vi "FormatLength.vi"(10 "length":i32) -> (2 "encoded length":string)   [LabVIEW 2014, in "Raspberry Pi Compatible Compiler for LabVIEW.lvlib" / "Websocket.lvlib"]
uses:
  Websocket.lvlib
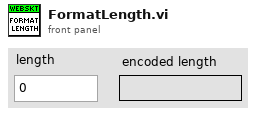
[diagram p1: front panel]
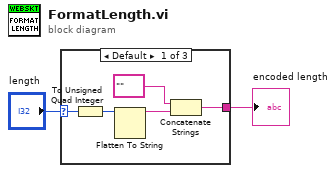
[diagram p0: block diagram]
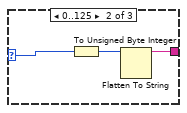
[diagram p2: hidden frame]
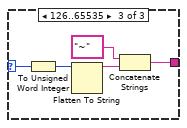
[diagram p3: hidden frame]
diagram:
  n1 = case shown="Default" "length" {
    selector: "length" -> [w7 w10 w15]
    tunnel: [w3 w8 w11] -> w1
    frame Default {
      n2 = To Unsigned Quad Integer(1:w7) -> (0:w6:u64)
      n3 = Flatten To String(anything=w6) -> (data string=w5:string)  [unwired: 3 in, 2 out]
      n4 = Concatenate Strings("", w5) -> (w3:string)
    }
    frame 0..125 {
      n5 = To Unsigned Byte Integer(number=w10) -> (unsigned 8bit integer=w9:u8)
      n6 = Flatten To String(anything=w9) -> (data string=w8:string)  [unwired: 3 in, 2 out]
    }
    frame 126..65535 {
      n7 = To Unsigned Word Integer(number=w15) -> (unsigned 16bit integer=w14:u16)
      n8 = Flatten To String(anything=w14) -> (data string=w13:string)  [unwired: 3 in, 2 out]
      n9 = Concatenate Strings("~", w13) -> (w11:string)
    }
  }
  "encoded length" <- w1
